vi "Ping Actors.vi"(8 "error in (no error)":errorcluster, 10 "Actor Core Name":string, 11 "Actor Monitor in":refnum<class "Actor Monitor.lvclass">) -> (0 "error out":errorcluster, 3 "Actor Monitor out":refnum<class "Actor Monitor.lvclass">)   [LabVIEW 2018, in "Monitored Actor.lvlib" / "Actor Monitor.lvclass"]
doc: "Sends a self addressed message to actor specified by the actor Core Name. If the Acotr Core Name is Empty, sends a poll message to every monitored Actor\n\nCopyright: MGI\nAuthored by: Derek Trepanier"
uses:
  Actor Monitor.lvclass
  C:/Program Files (x86)/National Instruments/LabVIEW 2018/vi.lib/ActorFramework/Actor/Actor.lvclass
  <vilib>/ActorFramework/Actor/Actor.lvclass/Actor.ctl
  <vilib>/ActorFramework/Message Enqueuer/Message Enqueuer.lvclass/Message Enqueuer.ctl
  Monitored Actor Messages/Ping Msg/Ping Msg.lvclass/Ping Msg.ctl
  <vilib>/ActorFramework/Message Enqueuer/Message Enqueuer.lvclass
  Actor Monitor.lvclass/Actor Monitor.ctl
  <vilib>/ActorFramework/Message Enqueuer/Init from Existing Queue.vi
  <vilib>/ActorFramework/Message Enqueuer/Enqueue.vi
  Monitored Actor Messages/Ping Msg/Ping Msg.lvclass
  C:/Program Files (x86)/National Instruments/LabVIEW 2018/vi.lib/ActorFramework/Message/Message.lvclass
  <vilib>/ActorFramework/Message Priority Queue/Priority Enqueue.vi
  <vilib>/ActorFramework/Actor/Actor.lvclass
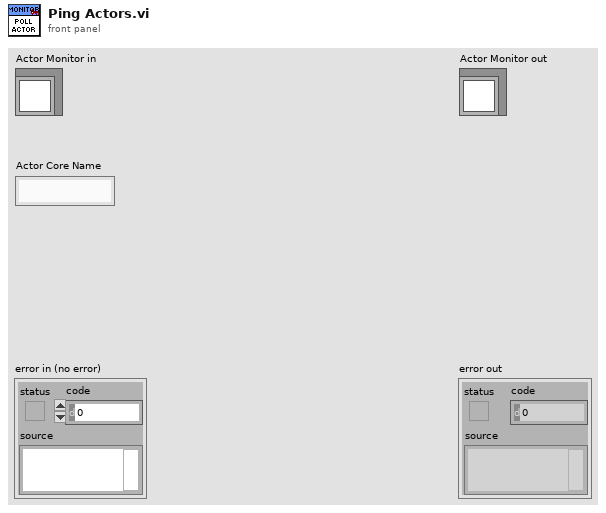
[diagram p1: front panel]
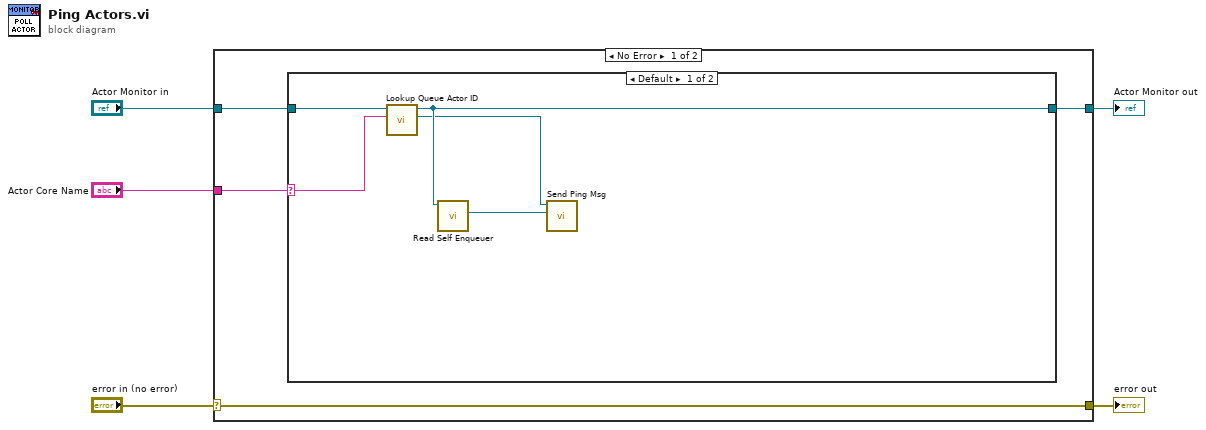
[diagram p0: block diagram]
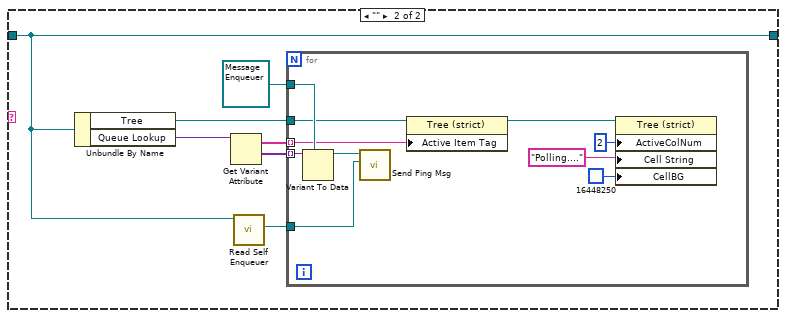
[diagram p2: hidden frame]
diagram:
  n1 = case shown="No Error" "error in (no error)" {
    selector: "error in (no error)" -> [w9 w33]
    tunnel: [w9 w33] -> w4
    tunnel: [w7 w32] -> w2
    tunnel: "Actor Monitor in" -> [w8 w32]
    tunnel: "Actor Core Name" -> [w6 _]
    frame No Error {
      n2 = case shown="Default" w6 {
        selector: w6 -> [w13 _]
        tunnel: w8 -> [w14 w18]
        tunnel: [w12 w18] -> w7
        frame Default {
          n3 = call "Lookup Queue Actor ID.vi"("Actor ID"=w13, "Actor Monitor in"=w14) -> ("Actor's Queue"=w11:refnum<class "Message Enqueuer.lvclass">, "Actor Monitor out"=w12:refnum<class "Actor Monitor.lvclass">)  [unwired: 7 in, 1 out]
          n4 = call <vilib>:"Read Self Enqueuer.vi"("Actor"=w12) -> ("Self Enqueuer"=w10:refnum<class "Message Enqueuer.lvclass">)  [unwired: 10 in]
          n5 = call "Send Ping Msg.vi"("Response Queue"=w10, "Message Enqueuer"=w11) -> ()  [unwired: 8 in, 2 out]
        }
        frame "" {
          n6 = Unbundle By Name(w18) -> ("Tree"=w16:refnum<vi>, "Queue Lookup"=w21:variant)
          n7 = Get Variant Attribute(Variant=w21) -> (names=w15:string[], values=w20:variant[])  [unwired: 3 in, 2 out]
          n8 = call <vilib>:"Read Self Enqueuer.vi"("Actor"=w18) -> ("Self Enqueuer"=w17:refnum<class "Message Enqueuer.lvclass">)  [unwired: 10 in]
          n9 = for {
            tunnel: w20 -> [w31] mode=indexing
            tunnel: refnum<class "Message Enqueuer.lvclass"> refnum ("Message Enqueuer") -> [w30]
            tunnel: w17 -> [w28]
            tunnel: w16 -> [w25]
            tunnel: w15 -> [w24] mode=indexing
            n10 = Variant To Data(type=w30, Variant=w31) -> (data=w29:refnum<class "Message Enqueuer.lvclass">)  [unwired: 1 in, 1 out]
            n11 = call "Send Ping Msg.vi"("Response Queue"=w28, "Message Enqueuer"=w29) -> ()  [unwired: 8 in, 2 out]
            n12 = property class="Tree (strict)"(reference=w25, "Active Item Tag"=w24) -> (reference out=w27:refnum<vi>)  [unwired: 1 in, 1 out]
            n13 = property class="Tree (strict)"(reference=w27, "ActiveColNum"=2 ("Active Cell:Active Column Number"), "Cell String"="Polling...." ("Active Cell:String"), "CellBG"=u32 16448250) -> ()  [unwired: 1 in, 2 out]
          }
        }
      }
    }
    frame Error {
    }
  }
  "error out" <- w4
  "Actor Monitor out" <- w2
